vi "Main.vi"(8 "error in":errorcluster, 9 "Error Queue":refnum<queue>, 11 "Application Events":refnum<user-event>) -> (0 "error out":errorcluster)   [LabVIEW 2020, in "Controller.lvlib"]
doc: "VI Template with default error structure"
uses:
  Controller.lvlib
  Error/Controls/Error Message Object.ctl
  Controls/Application Modules.ctl
  Error/Controls/Error Commands.ctl
  Controls/Application Event Object.ctl
  Controls/Application Events.ctl
  Controls/Application State.ctl
  Controls/Display Console State.ctl
  Controls/User Console State.ctl
  Controls/Module Internal State.ctl
  Controls/Event Loop Data.ctl
  Controls/Operational Loop Data.ctl
  Controls/Operational Loop Message Object.ctl
  Controls/Operational Loop Commands.ctl
  Configuration Database/Configuration Database.lvlib
  Error/Error Handler.lvlib
panel:
  out "Application State":T1
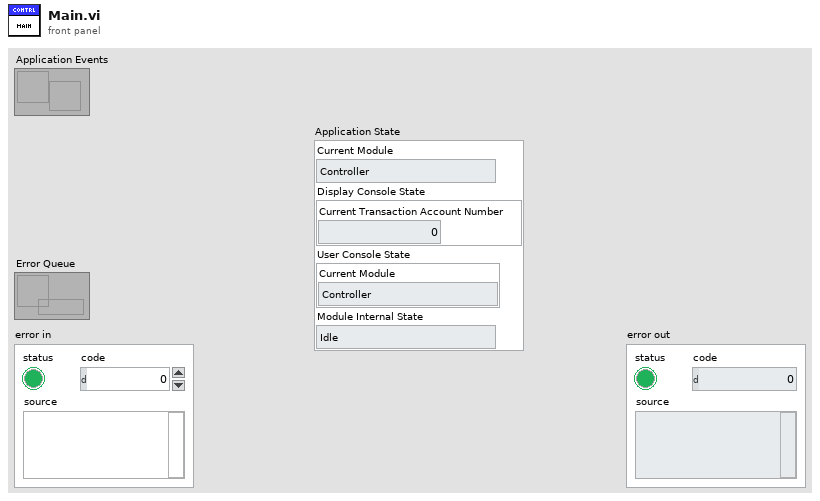
[diagram p1: front panel]
types:
  T1 = typedef "Controller.lvlib/Application State.ctl" = cluster{"Current Module":T2, "Display Console State":T3, "User Console State":T4, "Module Internal State":T5}
  T2 = typedef "Controller.lvlib/Application Modules.ctl" = enum16{"Controller", "Error Module", "User Console", "Display Console", "Sensor Interface"}
  T3 = typedef "Controller.lvlib/Display Console State.ctl" = cluster{"Current Transaction Account Number":i32}
  T4 = typedef "Controller.lvlib/User Console State.ctl" = cluster{"Current Module":T2}
  T5 = typedef "Controller.lvlib/Module Internal State.ctl" = enum16{"Idle"}
  T6 = typedef "Controller.lvlib/Operational Loop Message Object.ctl" = cluster{"Commands":T7, "Source Module":T2, "Event Data":variant}
  T7 = typedef "Controller.lvlib/Operational Loop Commands.ctl" = enum16{"Shutdown", "Initialize", "Time Target Reached", "Balance Enquiry", "Deposit", "Withdrawal", "Withdrawal: Amount", "Fast Cash $50", "New Transaction", "Terminate", "Idle", "Verify Account"}
  T8 = typedef "Controller.lvlib/Operational Loop Data.ctl" = cluster{"Attempt Number":i32}
  T9 = typedef "Controller.lvlib/Event Loop Data.ctl" = cluster{"Current Module":T2, "Timing":cluster{"isCounting":bool, "Timing Ticks Ms":i32, "Timing Target Sec":dbl, "Ticks Counter":i32}}
  T10 = typedef "Controller.lvlib/Application Events.ctl" = enum16{"Terminate App", "Initialize", "New Transaction", "Balance Inquiry", "Balance Inquiry: Answer", "Deposit", "Deposit: Answer", "Withdrawal", "Withdrawal: Amount", "Fast Cash 50$", "Terminate Session", "Login", "Verify Account", "Invalid Login"}
  T11 = enum16{"Load References", "Release References", "Get References"}
  T12 = typedef "Controller.lvlib/Application Event Object.ctl" = cluster{"Events":T10, "Source Module":T2, "Event Data":variant}
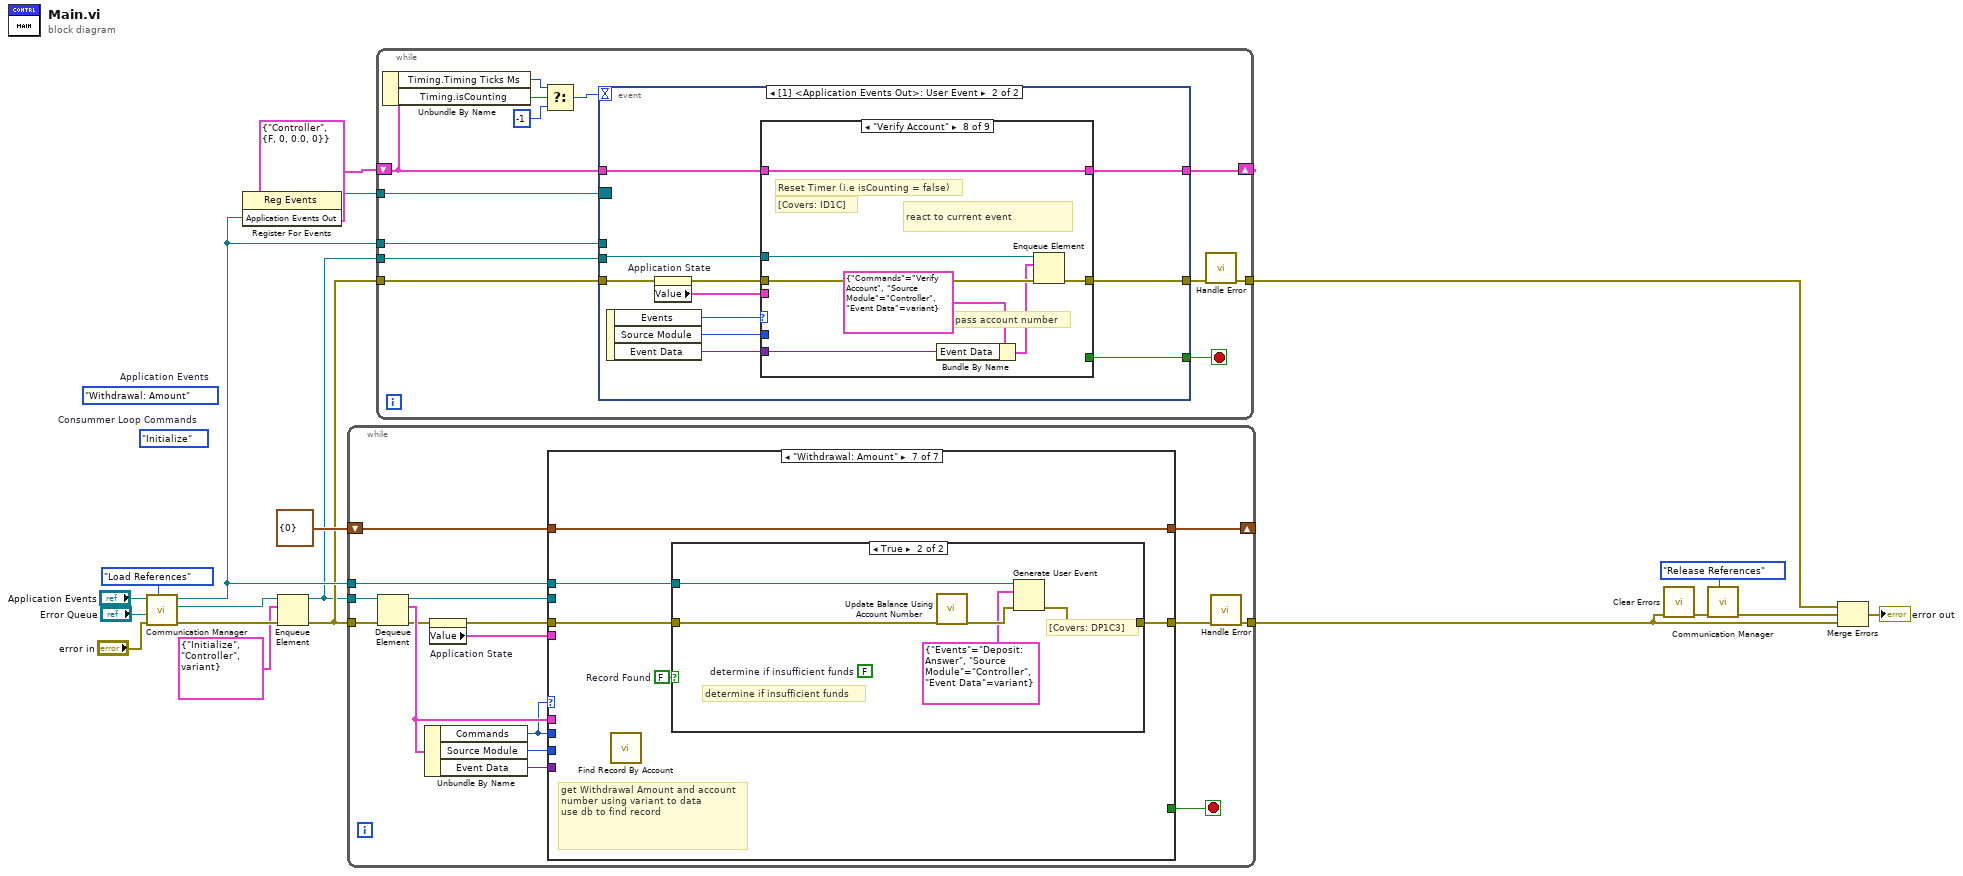
[diagram p0: block diagram]
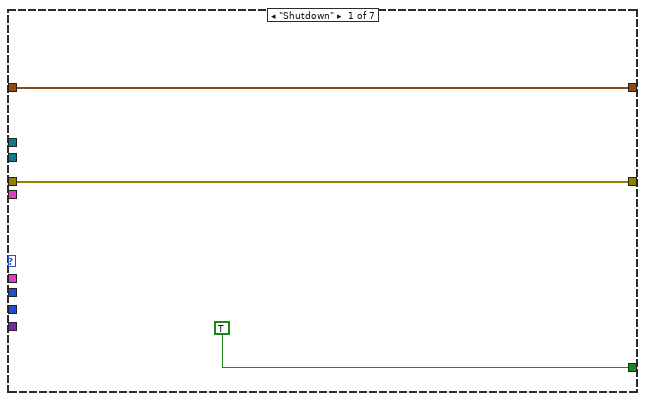
[diagram p2: hidden frame]
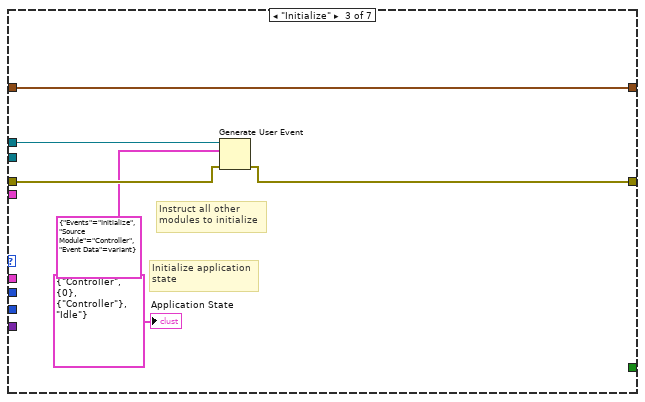
[diagram p4: hidden frame]
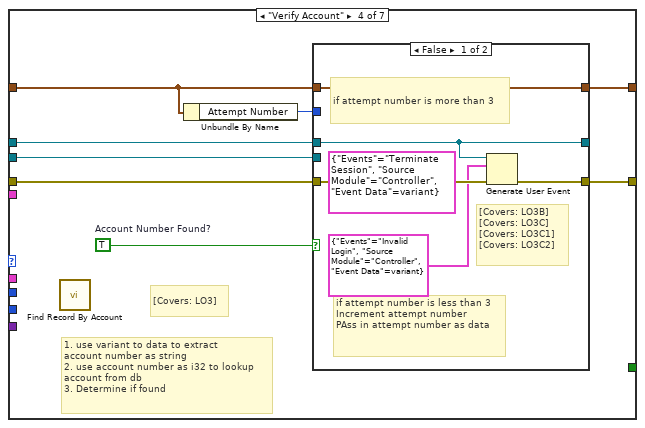
[diagram p5: hidden frame]
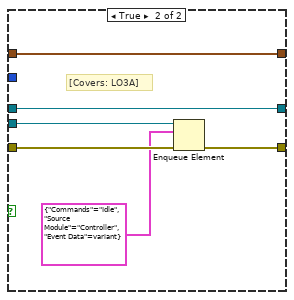
[diagram p6: hidden frame]
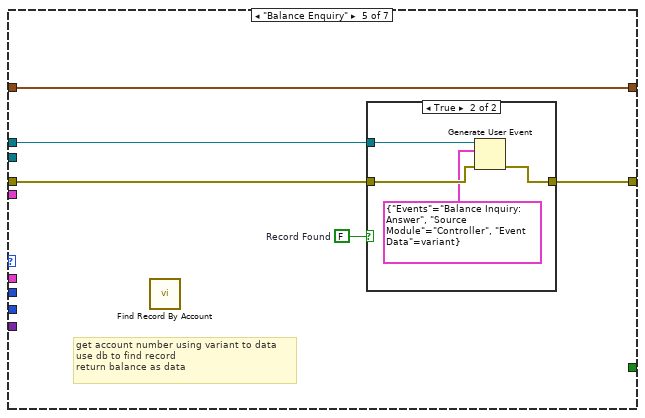
[diagram p7: hidden frame]
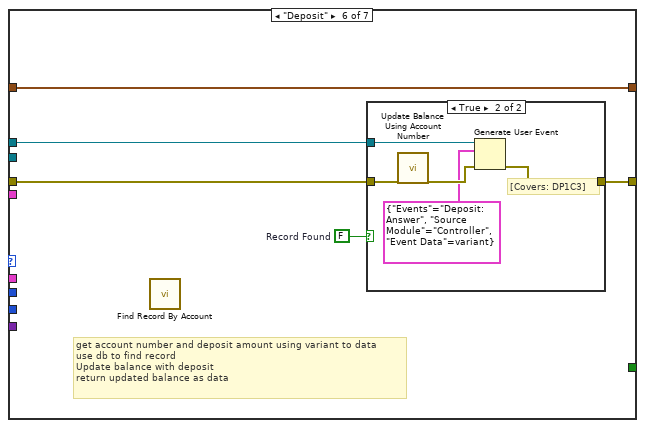
[diagram p9: hidden frame]
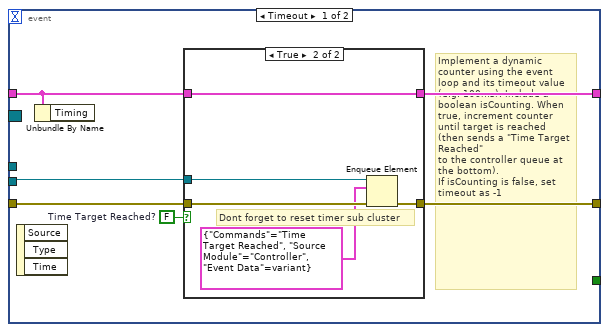
[diagram p12: hidden frame]
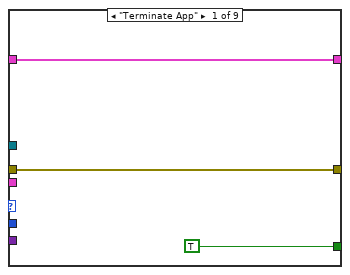
[diagram p14: hidden frame]
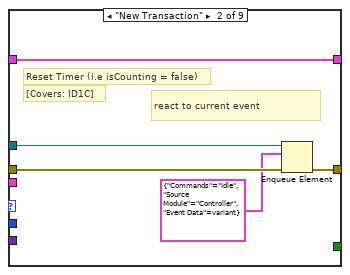
[diagram p15: hidden frame]
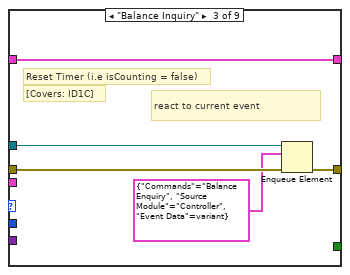
[diagram p16: hidden frame]
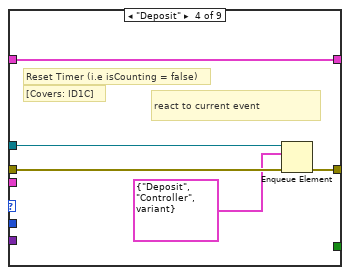
[diagram p17: hidden frame]
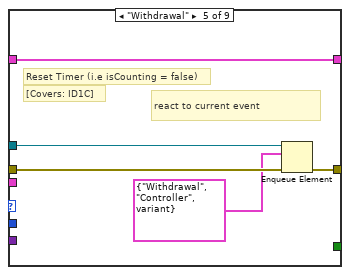
[diagram p18: hidden frame]
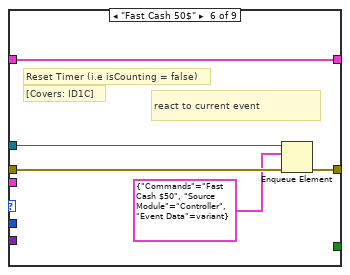
[diagram p19: hidden frame]
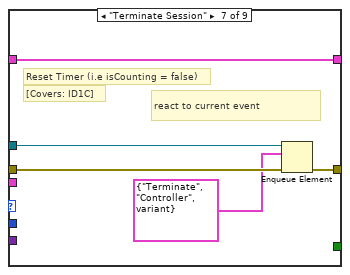
[diagram p20: hidden frame]
diagram:
  (unwired) Application_Events."Withdrawal: Amount"  # Application Events
  (unwired) Operational_Loop_Commands."Initialize"  # Consummer Loop Commands
  n1 = call "Communication Manager.vi"("Mode"=T11."Load References", "error in"="error in", "Error Queue"="Error Queue", "Application Events"="Application Events") -> ("error out"=w4:errorcluster, "Module Queue Out"=w3:refnum<queue>, "Application Events Out"=w8:refnum<user-event>)  [unwired: 4 in, 1 out]
  n2 = register-events(w8) -> (reference out=w7:refnum<event-registration>)  [unwired: 2 in, 1 out]
  n3 = Enqueue Element(queue=w3, element=T6 {"Commands"=enum."Initialize", "Source Module"=enum."Controller", "Event Data"=variant}, error in (no error)=w4) -> (queue out=w2:refnum<queue>)  [unwired: 1 in, 2 out]
  n4 = while {
    tunnel: w4 -> [w33]
    tunnel: w2 -> [w32]
    tunnel: [w34] -> w10
    tunnel: w8 -> [w25]
    shift-right: [w22] -> _
    shift-left: T8 {"Attempt Number"=0} ("Operational Loop Data") -> [w23]
    stop <- w26 stop-if-true
    n5 = Dequeue Element(queue=w32, error in (no error)=w33) -> (queue out=w24:refnum<queue>, element=w30:T6, error out=w21:errorcluster)  [unwired: 1 in, 1 out]
    n6 = Unbundle By Name(w30) -> ("Commands"=w27:T7, "Source Module"=w29:T2, "Event Data"=w28:variant)
    n7 = property on="Application State" class="Clust (strict)"(error in=w21) -> (error out=w20:errorcluster, "Value"=w19:T1)  [unwired: 1 in, 1 out]
    n8 = case shown="\"Withdrawal: Amount\"" w27 {
      tunnel: w20 -> [w37 w39 w42 w50 w67 w77 w87]
      tunnel: [w37 w39 w41 w51 w68 w78 w88] -> w31
      tunnel: w30 -> [_ _ _ _ _ _ _]
      tunnel: w27 -> [_ _ _ _ _ _ _]
      tunnel: w29 -> [_ _ _ _ _ _ _]
      tunnel: w28 -> [_ _ _ _ _ _ _]
      tunnel: [TRUE _ _ _ _ _ _] -> w26
      tunnel: w25 -> [_ _ w43 w52 w65 w75 w85]
      tunnel: w24 -> [_ _ _ w46 _ _ _]
      tunnel: w23 -> [w35 w38 w45 w48 w69 w79 w89]
      tunnel: [w35 w38 w45 w49 w69 w79 w89] -> w22
      tunnel: w19 -> [_ _ _ _ _ _ _]
      frame "Shutdown" {
      }
      frame Default {
      }
      frame "Initialize" {
        # "Instruct all other\nmodules to initialize"
        # "Initialize application\nstate"
        n9 = Generate User Event(user event=w43, event data cluster=T12 {"Events"=enum."Initialize", "Source Module"=enum."Controller", "Event Data"=variant} ("event data"), error in=w42) -> (error out=w41:errorcluster)  [unwired: 1 in, 1 out]
        "Application State" <- T1 {"Current Module"=enum."Controller", "Display Console State"={"Current Transaction Account Number"=0}, "User Console State"={"Current Module"=enum."Controller"}, "Module Internal State"=enum."Idle"} ("Application State")
      }
      frame "Verify Account" {
        w53 = TRUE  # Account Number Found?
        # "[Covers: LO3]"
        # "1. use variant to data to extract\naccount number as string\n2. use account number as i32 to lookup\naccount from db\n3. Determine if found"
        n10 = call "Find Record By Account.vi"() -> ()  [unwired: 10 in, 2 out]
        n11 = Unbundle By Name(w48) -> ("Attempt Number"=w47:i32)
        n12 = case shown="False" w53 {
          tunnel: [w56 w64] -> _
          tunnel: w52 -> [w56 w64]
          tunnel: [w57 w60] -> w51
          tunnel: w50 -> [w58 w62]
          tunnel: [w54 w63] -> w49
          tunnel: w48 -> [w54 w63]
          tunnel: w47 -> [_ _]
          tunnel: w46 -> [_ w61]
          frame False {
            (unwired) T12 {"Events"=enum."Terminate Session", "Source Module"=enum."Controller", "Event Data"=variant} ("event data")
            # "[Covers: LO3B] \n[Covers: LO3C] \n[Covers: LO3C1] \n[Covers: LO3C2]"
            # "if attempt number is more than 3"
            # "if attempt number is less than 3\nIncrement attempt number\nPAss in attempt number as data"
            n13 = Generate User Event(user event=w56, event data cluster=T12 {"Events"=enum."Invalid Login", "Source Module"=enum."Controller", "Event Data"=variant} ("event data"), error in=w58) -> (error out=w57:errorcluster)  [unwired: 1 in, 1 out]
          }
          frame True {
            # "[Covers: LO3A]"
            n14 = Enqueue Element(queue=w61, element=T6 {"Commands"=enum."Idle", "Source Module"=enum."Controller", "Event Data"=variant}, error in (no error)=w62) -> (error out=w60:errorcluster)  [unwired: 1 in, 2 out]
          }
        }
      }
      frame "Balance Enquiry" {
        w66 = FALSE  # Record Found
        # "get account number using variant to data\nuse db to find record\nreturn balance as data"
        n15 = call "Find Record By Account.vi"() -> ()  [unwired: 10 in, 2 out]
        n16 = case shown="True" w66 {
          tunnel: [w70 w73] -> w68
          tunnel: w67 -> [w70 w74]
          tunnel: w65 -> [_ w72]
          frame False {
            # "If not found, no response"
          }
          frame True {
            n17 = Generate User Event(user event=w72, event data cluster=T12 {"Events"=enum."Balance Inquiry: Answer", "Source Module"=enum."Controller", "Event Data"=variant} ("event data"), error in=w74) -> (error out=w73:errorcluster)  [unwired: 1 in, 1 out]
          }
        }
      }
      frame "Deposit" {
        w76 = FALSE  # Record Found
        # "get account number and deposit amount using variant to data\nuse db to find record\nUpdate balance with deposit\nreturn updated balance as data"
        n18 = call "Find Record By Account.vi"() -> ()  [unwired: 10 in, 2 out]
        n19 = case shown="True" w76 {
          tunnel: [w80 w83] -> w78
          tunnel: w77 -> [w80 w84]
          tunnel: w75 -> [_ w82]
          frame False {
            # "If not found, no response"
          }
          frame True {
            # "[Covers: DP1C3]"
            n20 = call "Update Balance Using Account Number.vi"() -> ()  [unwired: 10 in, 2 out]
            n21 = Generate User Event(user event=w82, event data cluster=T12 {"Events"=enum."Deposit: Answer", "Source Module"=enum."Controller", "Event Data"=variant} ("event data"), error in=w84) -> (error out=w83:errorcluster)  [unwired: 1 in, 1 out]
          }
        }
      }
      frame "Withdrawal: Amount" {
        w86 = FALSE  # Record Found
        # "get Withdrawal Amount and account number using variant to data\nuse db to find record"
        n22 = call "Find Record By Account.vi"() -> ()  [unwired: 10 in, 2 out]
        n23 = case shown="True" w86 {
          tunnel: [w90 w93] -> w88
          tunnel: w87 -> [w90 w94]
          tunnel: w85 -> [_ w92]
          frame False {
            # "If not found, no response"
          }
          frame True {
            (unwired) FALSE  # determine if insufficient funds
            # "determine if insufficient funds"
            # "[Covers: DP1C3]"
            n24 = call "Update Balance Using Account Number.vi"() -> ()  [unwired: 10 in, 2 out]
            n25 = Generate User Event(user event=w92, event data cluster=T12 {"Events"=enum."Deposit: Answer", "Source Module"=enum."Controller", "Event Data"=variant} ("event data"), error in=w94) -> (error out=w93:errorcluster)  [unwired: 1 in, 1 out]
          }
        }
      }
    }
    n26 = call "Handle Error.vi"("error in"=w31) -> ("error out"=w34:errorcluster)  [unwired: 10 in]
  }
  n27 = while {
    tunnel: w4 -> [w106]
    tunnel: w8 -> [w105]
    tunnel: [w107] -> w14
    tunnel: w2 -> [w104]
    tunnel: w7 -> [w103]
    shift-right: [w100] -> _
    shift-left: T9 {"Current Module"=enum."Controller", "Timing"={"isCounting"=FALSE, "Timing Ticks Ms"=0, "Timing Target Sec"=0.0, "Ticks Counter"=0}} ("Event Loop Data") -> [w99]
    stop <- w101 stop-if-true
    n28 = Unbundle By Name(w99) -> ("Timing.Timing Ticks Ms"=w97:i32, "Timing.isCounting"=w98:bool)
    n29 = Select(t=w97, s=w98, f=-1) -> (s? t:f=w95:i32)
    n30 = event shown="[1] <Application Events Out>: User Event" {
      selector: w103 -> [_ _]
      dyn-events: _ -> [_ _]
      timeout: w95 -> [_ _]
      tunnel: w106 -> [w113 w124]
      tunnel: w105 -> [_ _]
      tunnel: w104 -> [w112 w121]
      tunnel: [w111 w131] -> w102
      tunnel: [_ w127] -> w101
      tunnel: [w109 w126] -> w100
      tunnel: w99 -> [w108 w125]
      event Timeout {
        w110 = FALSE  # Time Target Reached?
        # "Implement a dynamic counter using the event\nloop and its timeout value (e.g. 100ms). Include a \nboolean isCounting. When true, increment counter\nuntil target is reached (then sends a \"Time Target Reached\"\nto the controller queue at the bottom).\nIf isCounting is false, set timeout as -1"
        n31 = event-data() -> ()  [unwired: 1 in, 3 out]
        n32 = Unbundle By Name(w108) -> ()  [unwired: 1 out]
        n33 = case shown="True" w110 {
          tunnel: w113 -> [w115 w120]
          tunnel: w112 -> [_ w119]
          tunnel: [w115 w118] -> w111
          tunnel: [w114 w116] -> w109
          tunnel: w108 -> [w114 w116]
          frame False {
          }
          frame True {
            # "Dont forget to reset timer sub cluster"
            n34 = Enqueue Element(queue=w119, element=T6 {"Commands"=enum."Time Target Reached", "Source Module"=enum."Controller", "Event Data"=variant}, error in (no error)=w120) -> (error out=w118:errorcluster)  [unwired: 1 in, 2 out]
          }
        }
      }
      event User Event {
        n35 = event-data() -> ("Events"=w130:T10, "Source Module"=w129:T2, "Event Data"=w128:variant)  [unwired: 1 in]
        n36 = property on="Application State" class="Clust (strict)"(error in=w124) -> (error out=w123:errorcluster, "Value"=w122:T1)  [unwired: 1 in, 1 out]
        n37 = case shown="\"Verify Account\"" w130 {
          tunnel: [w134 w137 w142 w147 w152 w157 w162 w169 w173] -> w131
          tunnel: w123 -> [w134 w138 w143 w148 w153 w158 w163 w170 w173]
          tunnel: w129 -> [_ _ _ _ _ _ _ _ _]
          tunnel: w128 -> [_ _ _ _ _ _ _ w165 _]
          tunnel: [TRUE _ _ _ _ _ _ _ _] -> w127
          tunnel: [w132 w139 w144 w149 w154 w159 w164 w171 w172] -> w126
          tunnel: w125 -> [w132 w139 w144 w149 w154 w159 w164 w171 w172]
          tunnel: w122 -> [_ _ _ _ _ _ _ _ _]
          tunnel: w121 -> [_ w136 w141 w146 w151 w156 w161 w168 _]
          frame "Terminate App" {
          }
          frame "New Transaction" {
            # "react to current event"
            # "[Covers: ID1C]"
            # "Reset Timer (i.e isCounting = false)"
            n38 = Enqueue Element(queue=w136, element=T6 {"Commands"=enum."Idle", "Source Module"=enum."Controller", "Event Data"=variant}, error in (no error)=w138) -> (error out=w137:errorcluster)  [unwired: 1 in, 2 out]
          }
          frame "Balance Inquiry" {
            # "react to current event"
            # "[Covers: ID1C]"
            # "Reset Timer (i.e isCounting = false)"
            n39 = Enqueue Element(queue=w141, element=T6 {"Commands"=enum."Balance Enquiry", "Source Module"=enum."Controller", "Event Data"=variant}, error in (no error)=w143) -> (error out=w142:errorcluster)  [unwired: 1 in, 2 out]
          }
          frame "Deposit" {
            # "react to current event"
            # "[Covers: ID1C]"
            # "Reset Timer (i.e isCounting = false)"
            n40 = Enqueue Element(queue=w146, element=T6 {"Commands"=enum."Deposit", "Source Module"=enum."Controller", "Event Data"=variant}, error in (no error)=w148) -> (error out=w147:errorcluster)  [unwired: 1 in, 2 out]
          }
          frame "Withdrawal" {
            # "react to current event"
            # "[Covers: ID1C]"
            # "Reset Timer (i.e isCounting = false)"
            n41 = Enqueue Element(queue=w151, element=T6 {"Commands"=enum."Withdrawal", "Source Module"=enum."Controller", "Event Data"=variant}, error in (no error)=w153) -> (error out=w152:errorcluster)  [unwired: 1 in, 2 out]
          }
          frame "Fast Cash 50$" {
            # "react to current event"
            # "[Covers: ID1C]"
            # "Reset Timer (i.e isCounting = false)"
            n42 = Enqueue Element(queue=w156, element=T6 {"Commands"=enum."Fast Cash $50", "Source Module"=enum."Controller", "Event Data"=variant}, error in (no error)=w158) -> (error out=w157:errorcluster)  [unwired: 1 in, 2 out]
          }
          frame "Terminate Session" {
            # "react to current event"
            # "[Covers: ID1C]"
            # "Reset Timer (i.e isCounting = false)"
            n43 = Enqueue Element(queue=w161, element=T6 {"Commands"=enum."Terminate", "Source Module"=enum."Controller", "Event Data"=variant}, error in (no error)=w163) -> (error out=w162:errorcluster)  [unwired: 1 in, 2 out]
          }
          frame "Verify Account" {
            # "pass account number"
            # "react to current event"
            # "[Covers: ID1C]"
            # "Reset Timer (i.e isCounting = false)"
            n44 = Bundle By Name(cluster=T6 {"Commands"=enum."Verify Account", "Source Module"=enum."Controller", "Event Data"=variant} ("element"), "Event Data"=w165) -> (w166:T6)
            n45 = Enqueue Element(queue=w168, element=w166, error in (no error)=w170) -> (error out=w169:errorcluster)  [unwired: 1 in, 2 out]
          }
          frame Default {
          }
        }
      }
    }
    n46 = call "Handle Error.vi"("error in"=w102) -> ("error out"=w107:errorcluster)  [unwired: 10 in]
  }
  n47 = call <vilib>:"Clear Errors.vi"("error in (no error)"=w10) -> ("error out"=w13:errorcluster)  [unwired: 5 in, 1 out]
  n48 = call "Communication Manager.vi"("Mode"=T11."Release References", "error in"=w13) -> ("error out"=w9:errorcluster)  [unwired: 6 in, 3 out]
  n49 = Merge Errors(w14, w9, w10) -> (→"error out":errorcluster)
